vi "Practica 17 - Sensor de temperatura.vi"() -> ()   [LabVIEW 2020]
panel:
  in  "stop":bool
  in  "Sensor":dbl(knob) scale=0.0..120.0
  out "Mensaje de Advertencia":string
  out "ERROR":bool
  out "Temp. Maxima":bool
  out "Temp. en Rango":bool
  out "Temp. Baja":bool
  out "Temp. sensada":dbl
  in  "Max. Temperatura":dbl
  in  "Min. Temperatura":dbl
  # "SENSOR DE TEMPERATURA"
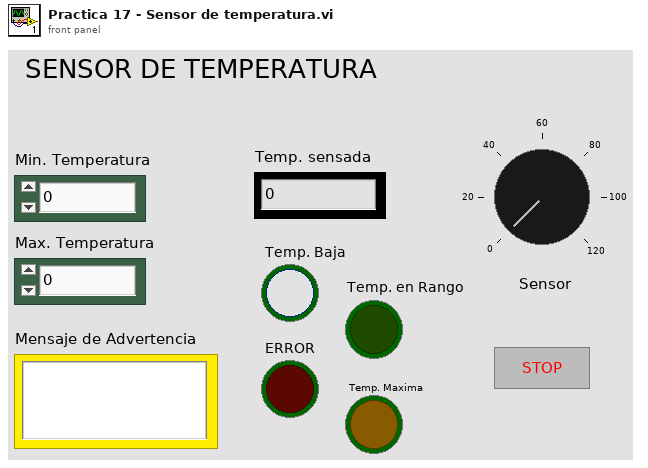
[diagram p1: front panel]
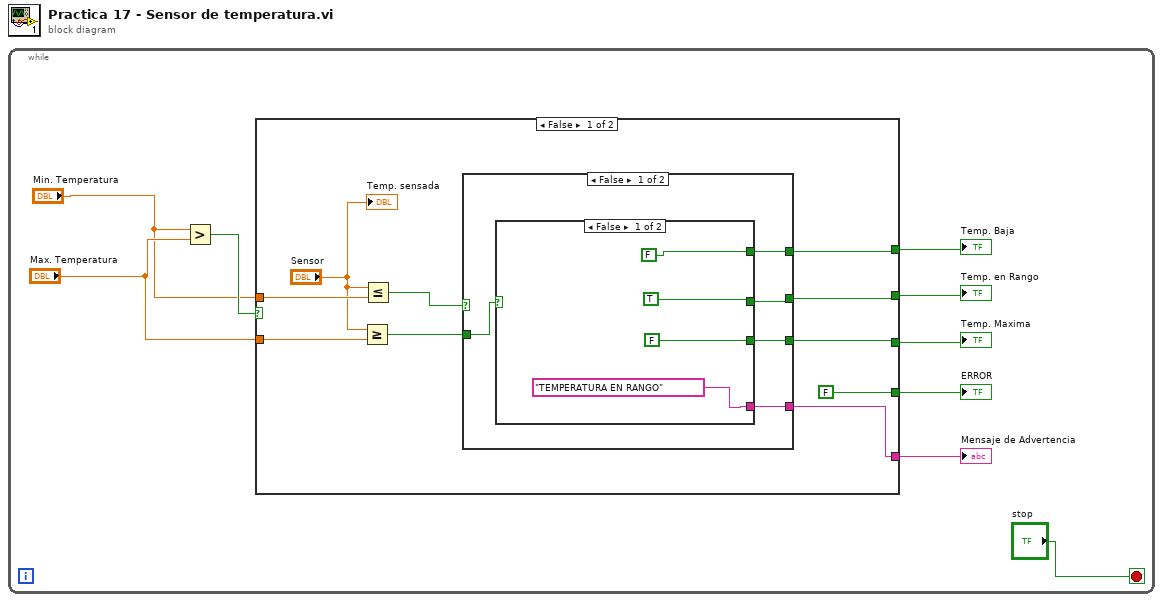
[diagram p0: block diagram]
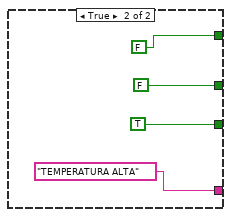
[diagram p2: hidden frame]
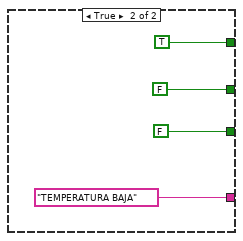
[diagram p3: hidden frame]
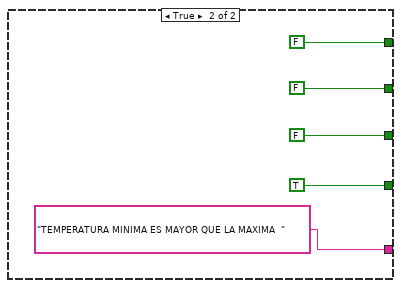
[diagram p4: hidden frame]
diagram:
  n1 = while {
    stop <- "stop" stop-if-true
    n2 = Greater?(x="Min. Temperatura", y="Max. Temperatura") -> (0:w9:bool)
    n3 = case shown="False" w9 {
      tunnel: [FALSE TRUE] -> w8
      tunnel: [w13 FALSE] -> w7
      tunnel: [w15 "TEMPERATURA MINIMA ES MAYOR QUE LA MAXIMA  "] -> w6
      tunnel: [w11 FALSE] -> w5
      tunnel: [w12 FALSE] -> w4
      tunnel: "Max. Temperatura" -> [w19 _]
      tunnel: "Min. Temperatura" -> [w18 _]
      frame False {
        n4 = Greater Or Equal?(x="Sensor", y=w19) -> (x >= y?=w10:bool)
        n5 = Less Or Equal?(x="Sensor", y=w18) -> (x <= y?=w14:bool)
        n6 = case shown="False" w14 {
          tunnel: [w23 "TEMPERATURA BAJA"] -> w15
          tunnel: [w20 TRUE] -> w13
          tunnel: [w22 FALSE] -> w12
          tunnel: [w21 FALSE] -> w11
          tunnel: w10 -> [w24 _]
          frame False {
            n7 = case shown="False" w24 {
              tunnel: ["TEMPERATURA EN RANGO" "TEMPERATURA ALTA"] -> w23
              tunnel: [FALSE TRUE] -> w22
              tunnel: [TRUE FALSE] -> w21
              tunnel: [FALSE FALSE] -> w20
              frame False {
              }
              frame True {
              }
            }
          }
          frame True {
          }
        }
        "Temp. sensada" <- "Sensor"
      }
      frame True {
      }
    }
    "Temp. Baja" <- w7
    "Temp. en Rango" <- w5
    "Temp. Maxima" <- w4
    "ERROR" <- w8
    "Mensaje de Advertencia" <- w6
  }
